vi "LE 8 Byte Array to fp64 (Subvi).vi"(9 "8 Bytes in":u8[](array[numeric])) -> (3 "fp64 Out":dbl)   [LabVIEW 2019]
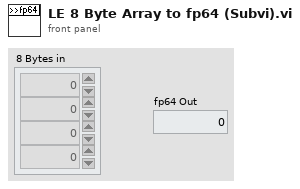
[diagram p1: front panel]
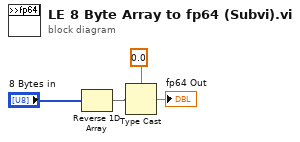
[diagram p0: block diagram]
diagram:
  n1 = Reverse 1D Array(array="8 Bytes in") -> (reversed array=w4:u8[])
  n2 = Type Cast(type=0.0, x=w4) -> (*(type *) &x=→"fp64 Out":dbl)
